vi "Rationalize number.vi"(11 "number in":dbl) -> (3 "rationalized":cluster{"n":u64, "d":u64})   [LabVIEW 2018, in "GettingStarted_5785_Host.lvlib"]
uses:
  GettingStarted_5785_Host.lvlib
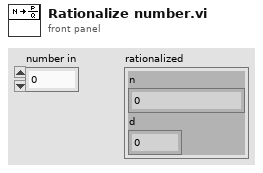
[diagram p1: front panel]
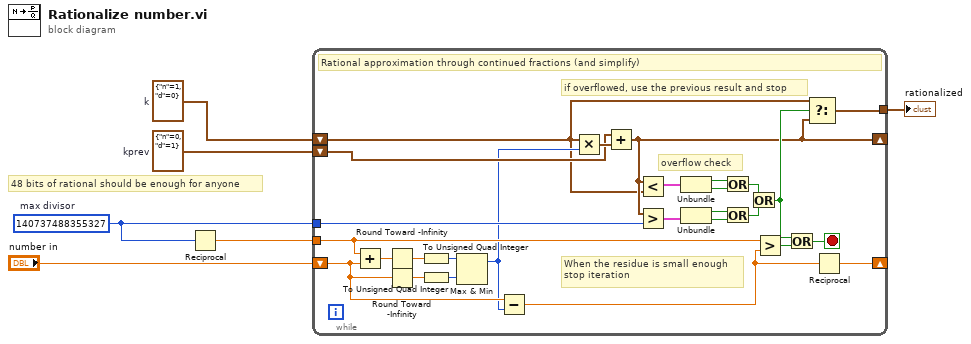
[diagram p0: block diagram]
diagram:
  w6 = cluster{"n":u64, "d":u64} {"n"=0, "d"=1}  # kprev
  w4 = u64 140737488355327  # max divisor
  w2 = cluster{"n":u64, "d":u64} {"n"=1, "d"=0}  # k
  # "48 bits of rational should be enough for anyone"
  n1 = Reciprocal(x=w4) -> (1/x=w1:dbl)
  n2 = while {
    tunnel: w1 -> [w23]
    shift-right: [w10] -> _
    shift-left: w2 -> [w9]
    shift-right: [w15] -> _
    shift-left: "number in" -> [w14]
    shift-left: w6 -> [w13]
    tunnel: [w22] -> w5
    tunnel: w4 -> [w18]
    stop <- w21 stop-if-true
    # "if overflowed, use the previous result and stop"
    # "When the residue is small enough\nstop iteration"
    # "overflow check"
    # "Rational approximation through continued fractions (and simplify)"
    n3 = Add(x=w23, y=w14) -> (x+y=w33:dbl)
    n4 = Round Toward -Infinity(1:w33) -> (0:w8:dbl)
    n5 = Round Toward -Infinity(1:w14) -> (0:w7:dbl)
    n6 = To Unsigned Quad Integer(1:w8) -> (0:w32:u64)
    n7 = To Unsigned Quad Integer(1:w7) -> (0:w12:u64)
    n8 = Max & Min(x=w32, y=w12) -> (max(x,y)=w11:u64)  [unwired: 1 out]
    n9 = Subtract(x=w14, y=w11) -> (x-y=w16:dbl)
    n10 = Multiply(x=w9, y=w11) -> (x*y=w31:cluster{"n":u64, "d":u64})
    n11 = Add(x=w13, y=w31) -> (x+y=w10:cluster{"n":u64, "d":u64})
    n12 = Less?(x=w10, y=w9) -> (x < y?=w30:cluster{"n":bool, "d":bool})
    n13 = Greater?(x=w10, y=w18) -> (0:w25:cluster{"n":bool, "d":bool})
    n14 = Unbundle(w30) -> ("n"=w29:bool, "d"=w28:bool)
    n15 = Unbundle(w25) -> ("n"=w26:bool, "d"=w27:bool)
    n16 = Or(x=w29, y=w28) -> (x .or. y?=w24:bool)
    n17 = Or(x=w26, y=w27) -> (x .or. y?=w17:bool)
    n18 = Or(x=w24, y=w17) -> (x .or. y?=w20:bool)
    n19 = Greater?(x=w23, y=w16) -> (0:w19:bool)
    n20 = Or(x=w20, y=w19) -> (x .or. y?=w21:bool)
    n21 = Select(t=w9, s=w20, f=w10) -> (s? t:f=w22:cluster{"n":u64, "d":u64})
    n22 = Reciprocal(x=w16) -> (1/x=w15:dbl)
  }
  "rationalized" <- w5
